vi "Master network read write.vi"(7 "Modbus master in":refnum<class "Modbus Master.lvclass">, 8 "error in":errorcluster, 9 "transmission data unit in":refnum<class "Transmission Data Unit.lvclass">, 10 "network master in":refnum<class "Network Master.lvclass">, 11 "Modbus data unit in":refnum<class "Modbus Data Unit.lvclass">) -> (0 "error out":errorcluster, 2 "PDU Valid?":bool, 3 "Modbus data unit out":refnum<class "Modbus Data Unit.lvclass">, 5 "Modbus master out":refnum<class "Modbus Master.lvclass">)   [LabVIEW 2014, in "MyLib.lvlib" / "Modbus Master.lvclass"]
doc: "This VI allows a mutex for the master API without restricting any other functions. This mutex is currently unimplemented."
uses:
  Modbus Master.lvclass
  Network Protocol/Network Master/Network Master.lvclass
  Transmission Data Unit/Transmission Data Unit.lvclass
  Modbus Data Unit/Modbus Data Unit.lvclass
  Modbus Master.lvclass/Modbus Master.ctl
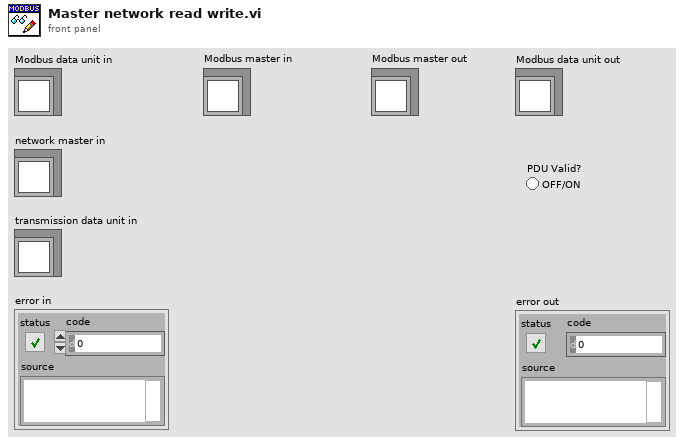
[diagram p1: front panel]
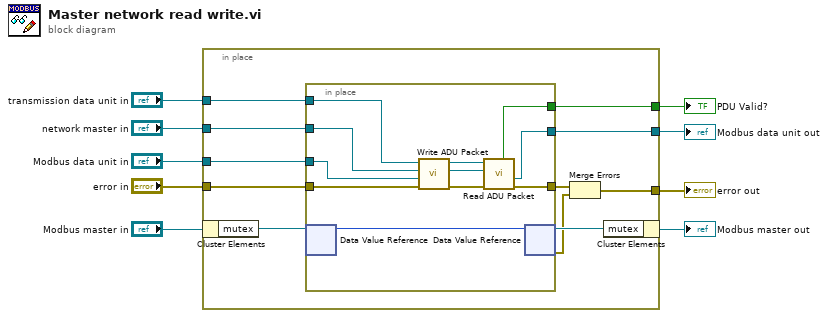
[diagram p0: block diagram]
diagram:
  n1 = in-place {
    in-place-border: "error in" -> [w19]
    in-place-border: "Modbus data unit in" -> [w18]
    in-place-border: "transmission data unit in" -> [w16]
    in-place-border: "network master in" -> [w15]
    in-place-border: [w12] -> w3
    in-place-border: [w11] -> w2
    in-place-border: [w10] -> w1
    n2 = in-place-cluster #1("Modbus master in") -> ("mutex"=w20:refnum<data-value>)
    n3 = in-place {
      in-place-border: w19 -> [w27]
      in-place-border: w18 -> [w26]
      in-place-border: w16 -> [w25]
      in-place-border: w15 -> [w23]
      in-place-border: [w24] -> w14
      in-place-border: [w22] -> w12
      in-place-border: [w21] -> w10
      n4 = in-place-dvr #2(w20) -> (w28:u8)  [unwired: 1 out]
      n5 = call-dynamic "Write ADU Packet.vi"("error in"=w27, "modbus data unit"=w26, "protocol layer"=w23, "transmission data unit in"=w25) -> ("error out"=w30:errorcluster, "protocol layer out"=w31:refnum<class "Network Protocol.lvclass">, "transmission data unit out"=w29:refnum<class "Transmission Data Unit.lvclass">)  [unwired: 5 in]
      n6 = call-dynamic "Read ADU Packet.vi"("error in"=w30, "protocol layer"=w31, "transmission data unit in"=w29) -> ("error out"=w24:errorcluster, "modbus data unit"=w22:refnum<class "Modbus Data Unit.lvclass">, "PDU Valid?"=w21:bool)  [unwired: 4 in, 2 out]
      n7 = in-place-dvr #2(w28) -> (w17:refnum<data-value>, w13:errorcluster)
    }
    n8 = Merge Errors(w14, w13) -> (w11:errorcluster)
    n9 = in-place-cluster #1("mutex"=w17) -> (→"Modbus master out":refnum<class "Modbus Master.lvclass">)
  }
  "Modbus data unit out" <- w3
  "error out" <- w2
  "PDU Valid?" <- w1
